vi "Timestamp_Converter.vi"(7 "Date String":string, 8 "Date":timestamp format="%<%x>T") -> (1 "Date":timestamp format="%<%x>T", 2 "Date string":string)   [LabVIEW 2024]
panel:
  out "error out":errorcluster
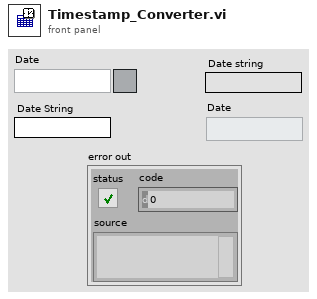
[diagram p1: front panel]
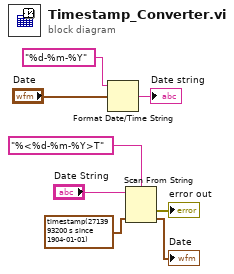
[diagram p0: block diagram]
diagram:
  n1 = Format Date/Time String(time format string (%c)="%d-%m-%Y" ("format string"), seconds (now)="Date") -> (date/time string=→"Date string":string)  [unwired: 1 in]
  n2 = Scan From String(format string="%<%d-%m-%Y>T", input string="Date String", default 1=timestamp(2713993200 s since 1904-01-01) ("default value 1")) -> (error out=→"error out":errorcluster, output 1=→"Date":timestamp)  [unwired: 2 in, 2 out]
